vi "Read DXF File.vi"(0 "path":path, 11 "error in (no error)":errorcluster) -> (4 "XY graph":cluster{dbl[], dbl[]}[](array[cluster]), 15 "error out":errorcluster)   [LabVIEW 2020, in "Graph Module.lvlib"]
uses:
  Graph Module.lvlib
  D:/Git/netDxf_2.4.2/bin/Release/netDxf.dll
  netDxf_2.4.2/bin/Release/netDxf.dll
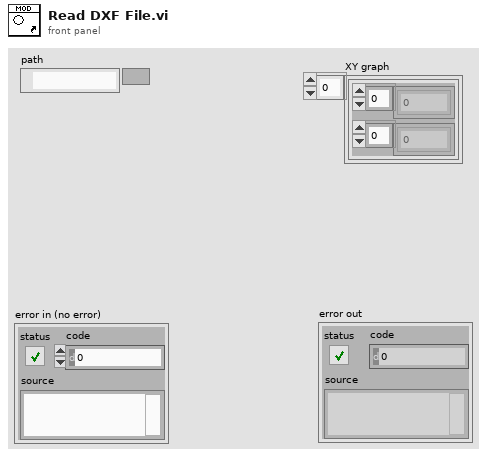
[diagram p1: front panel]
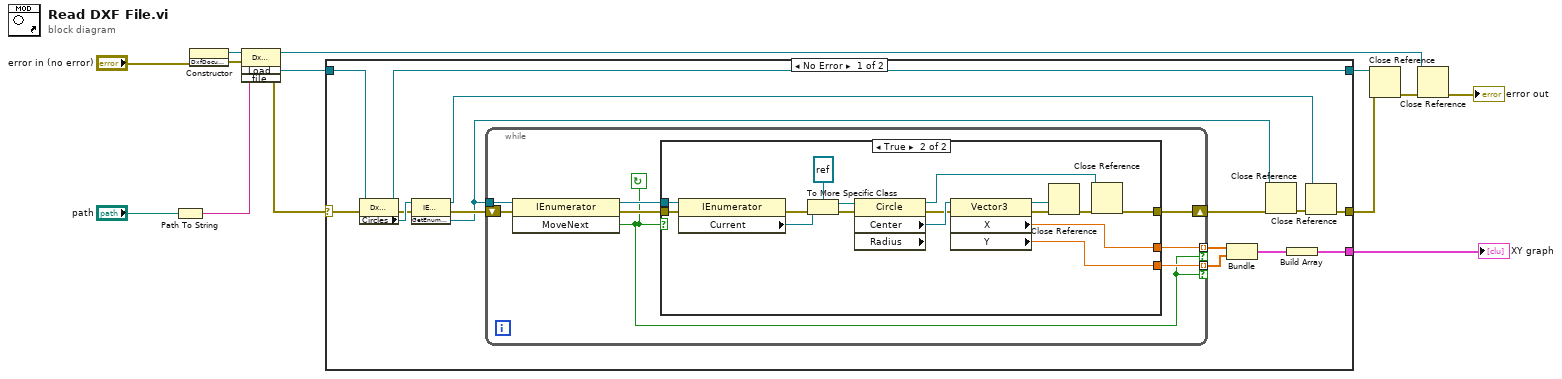
[diagram p0: block diagram]
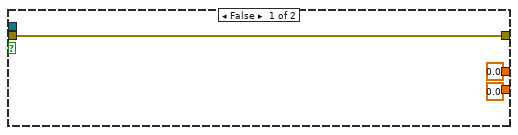
[diagram p2: hidden frame]
diagram:
  n1 = Path To String(path="path") -> (string=w12:string)
  n2 = constructor class="DxfDocument"(error in="error in (no error)") -> (reference out=w1:refnum<k24>, error out=w13:errorcluster)  [unwired: 2 in, 1 out]
  n3 = invoke class="DxfDocument" method="Load"(reference=w1, error in=w13, "file"=w12) -> (reference out=w9:refnum<k24>, error out=w7:errorcluster, "Load"=w8:refnum<k24>)  [unwired: 1 in, 1 out]
  n4 = case shown="No Error" w7 {
    selector: w7 -> [w18 w57]
    tunnel: w8 -> [w25 w56]
    tunnel: [w24 w56] -> w11
    tunnel: [w19 w57] -> w4
    tunnel: [w14 _] -> w2
    frame No Error {
      n5 = property class="DxfDocument"(reference=w25, error in=w18) -> (reference out=w24:refnum<k24>, error out=w26:errorcluster, "Circles"=w28:refnum<k24>)
      n6 = invoke class="IEnumerable`1[[netDxf.Entities." method="GetEnumerator"(reference=w28, error in=w26) -> (reference out=w20:refnum<k24>, error out=w27:errorcluster, "GetEnumerator"=w23:refnum<k24>)  [unwired: 1 in]
      n7 = while {
        tunnel: [w31] -> w17 mode=indexing if=w29
        tunnel: w23 -> [w33]
        shift-right: [w36] -> w22
        shift-left: w27 -> [w32]
        tunnel: [w30] -> w16 mode=indexing if=w29
        stop <- w29 continue-if-true
        n8 = invoke class="IEnumerator" method="MoveNext"(reference=w33, error in=w32) -> (reference out=w35:refnum<k24>, error out=w34:errorcluster, "MoveNext"=w29:bool)  [unwired: 1 in]
        n9 = case shown="True" w29 {
          tunnel: [w39 w55] -> w36
          tunnel: w35 -> [_ w43]
          tunnel: w34 -> [w39 w42]
          tunnel: [0.0 ("X") w41] -> w31
          tunnel: [0.0 ("Y") w40] -> w30
          frame False {
          }
          frame True {
            n10 = property class="IEnumerator"(reference=w43, error in=w42) -> (error out=w44:errorcluster, "Current"=w45:refnum<k24>)  [unwired: 1 out]
            n11 = To More Specific Class(target class=refnum<k24> refnum ("new reference"), reference=w45, error in=w44) -> (specific class reference=w53:refnum<k24>, error out=w50:errorcluster)
            n12 = property class="Circle" props=["Center", "Radius"](reference=w53, error in=w50) -> (reference out=w47:refnum<k24>, error out=w51:errorcluster, "Center"=w52:refnum<k24>)  [unwired: 1 out]
            n13 = property class="Vector3"(reference=w52, error in=w51) -> (reference out=w49:refnum<k24>, error out=w48:errorcluster, "X"=w41:dbl, "Y"=w40:dbl)
            n14 = Close Reference(reference=w49, error in (no error)=w48) -> (error out=w46:errorcluster)
            n15 = Close Reference(reference=w47, error in (no error)=w46) -> (error out=w55:errorcluster)
          }
        }
      }
      n16 = Bundle(w17, w16) -> (w15:cluster{dbl[], dbl[]})  [unwired: 1 in]
      n17 = Close Reference(reference=w23, error in (no error)=w22) -> (error out=w21:errorcluster)
      n18 = Build Array(w15) -> (w14:cluster{dbl[], dbl[]}[])
      n19 = Close Reference(reference=w20, error in (no error)=w21) -> (error out=w19:errorcluster)
    }
    frame Error {
    }
  }
  "XY graph" <- w2
  n20 = Close Reference(reference=w11, error in (no error)=w4) -> (error out=w10:errorcluster)
  n21 = Close Reference(reference=w9, error in (no error)=w10) -> (error out=→"error out":errorcluster)
